vi "Calculate possible moves.vi"(8 "error in (no error)":errorcluster, 11 "Position in":refnum<class "Position.lvclass">) -> (0 "error out":errorcluster, 2 "Moves":refnum<class "Move.lvclass">[](array[class]), 3 "Position out":refnum<class "Position.lvclass">)   [LabVIEW 2016, in "Chesslib.lvlib" / "Position.lvclass"]
uses:
  Position.lvclass
  Moves/Move/Move.lvclass
  Position.lvclass/Position.ctl
  Pieces/Piece/Piece.lvclass
  Board/Board.lvclass
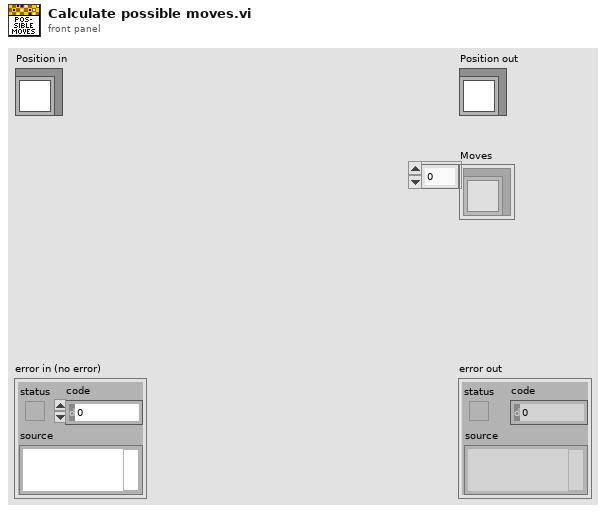
[diagram p1: front panel]
types:
  T1 = typedef "Chesslib.lvlib/Color.ctl" = enum16{"White", "Black"}
  T2 = typedef "Chesslib.lvlib/Square.ctl" = cluster{"File":T3, "Rank":T4}
  T3 = typedef "Chesslib.lvlib/File.ctl" = enum8{"a", "b", "c", "d", "e", "f", "g", "h"}
  T4 = typedef "Chesslib.lvlib/Rank.ctl" = enum8{"1", "2", "3", "4", "5", "6", "7", "8"}
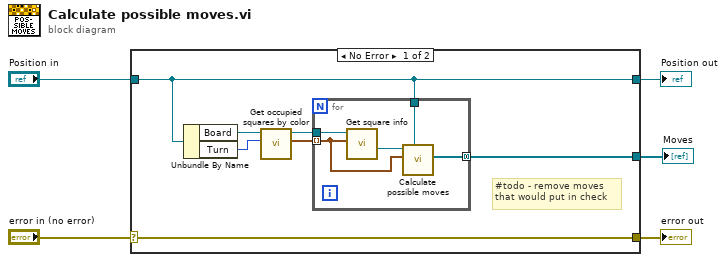
[diagram p0: block diagram]
diagram:
  n1 = case shown="No Error" "error in (no error)" {
    selector: "error in (no error)" -> [w12 w19]
    tunnel: [w12 w19] -> w4
    tunnel: [w7 w18] -> w2
    tunnel: "Position in" -> [w7 w18]
    tunnel: [w6 _] -> w1
    frame No Error {
      # "#todo - remove moves\nthat would put in check"
      n2 = Unbundle By Name(w7) -> ("Board"=w11:refnum<class "Board.lvclass">, "Turn"=w10:T1)
      n3 = call "Get occupied squares by color.vi"("Color"=w10, "Board in"=w11) -> ("Squares"=w9:T2[], "Board out"=w8:refnum<class "Board.lvclass">)  [unwired: 8 in]
      n4 = for {
        tunnel: w9 -> [w14] mode=indexing
        tunnel: w8 -> [w17]
        tunnel: w7 -> [w15]
        tunnel: [w13] -> w6 mode=concatenating
        n5 = call "Get square info.vi"("Square"=w14, "Board in"=w17) -> ("Piece"=w16:refnum<class "Piece.lvclass">)  [unwired: 7 in, 2 out]
        n6 = call-dynamic "Calculate possible moves.vi"("Position"=w15, "Source"=w14, "Piece in"=w16) -> ("Moves"=w13:refnum<class "Move.lvclass">[])  [unwired: 6 in, 2 out]
      }
    }
    frame Error {
    }
  }
  "error out" <- w4
  "Position out" <- w2
  "Moves" <- w1
